vi "Poll Home Control.vi"(8 "error in (no error)":errorcluster, 11 "Cylinder.lvclass":refnum<class "Cylinder.lvclass">) -> ()   [LabVIEW 2015, in "cRIO-Carbondioxide.lvlib" / "CO2-Actor.lvlib" / "Cylinder.lvclass"]
uses:
  Cylinder.lvclass
  Cylinder.lvclass/Cylinder.ctl
  <vilib>/ActorFramework/Actor/Actor.lvclass/Actor.ctl
  <vilib>/ActorFramework/Message Enqueuer/Message Enqueuer.lvclass/Message Enqueuer.ctl
  Cylinder Messages/Run Msg/Run Msg.lvclass/Run Msg.ctl
  Cylinder Messages/Home Msg/Home Msg.lvclass/Home Msg.ctl
  <vilib>/ActorFramework/Actor/Read Self Enqueuer.vi
  <vilib>/ActorFramework/Message Enqueuer/Enqueue.vi
  <vilib>/ActorFramework/Message Enqueuer/Init from Existing Queue.vi
  <vilib>/ActorFramework/Message Priority Queue/Priority Enqueue.vi
  <vilib>/ActorFramework/Actor/Actor.lvclass
  <vilib>/ActorFramework/Message Enqueuer/Message Enqueuer.lvclass
  Interlocks/Interlock Chain/Interlock Chain.lvclass
  Cylinder Messages/Run Msg/Run Msg.lvclass
  Cylinder Messages/Home Msg/Home Msg.lvclass
  cRIO-CO2/cRIO-CO2.lvclass
  CO2 Actor/CO2 Actor.lvclass
panel:
  out "error out":errorcluster
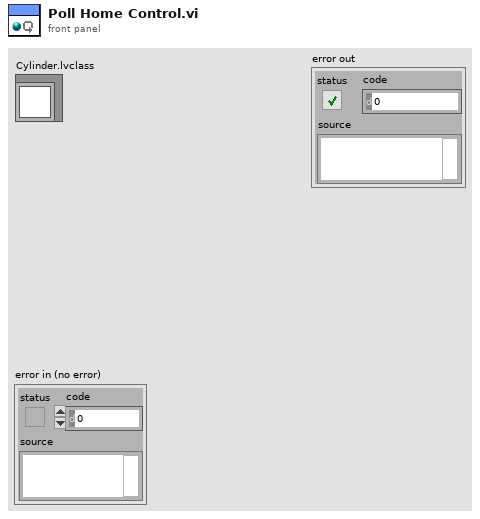
[diagram p1: front panel]
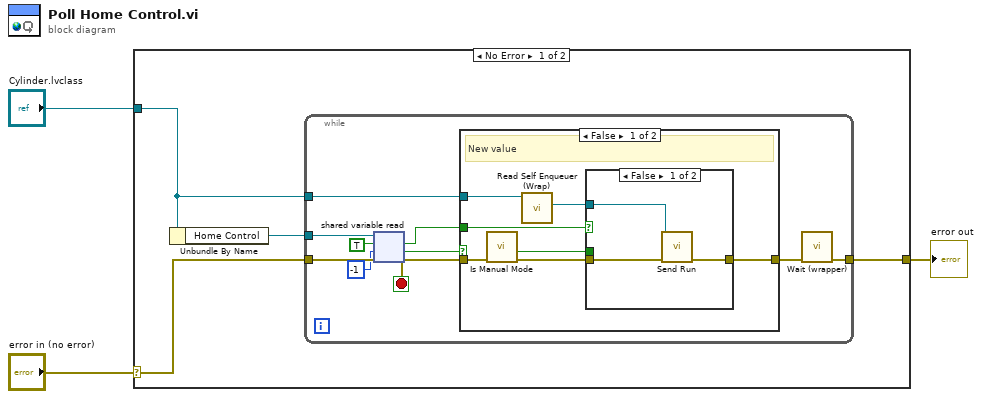
[diagram p0: block diagram]
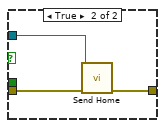
[diagram p2: hidden frame]
diagram:
  n1 = case shown="No Error" "error in (no error)" {
    selector: "error in (no error)" -> [w5 w32]
    tunnel: "Cylinder.lvclass" -> [w6 _]
    tunnel: [w4 w32] -> w1
    frame No Error {
      n2 = Unbundle By Name(w6) -> ("Home Control"=w7:refnum<k21>)
      n3 = while {
        tunnel: w7 -> [w17]
        tunnel: w5 -> [w16]
        tunnel: w6 -> [w10]
        tunnel: [w8] -> w4
        stop <- w11 stop-if-true
        n4 = shared-variable-read(w17, w16, TRUE, -1 ("timeout ms")) -> (w11:errorcluster, w9:bool, w12:bool)  [unwired: 2 out]
        n5 = case shown="False" w9 {
          tunnel: w12 -> [w21 _]
          tunnel: [w22 w31] -> w13
          tunnel: w11 -> [w24 w31]
          tunnel: w10 -> [w19 _]
          frame False {
            # "New value"
            n6 = call "Is Manual Mode.vi"("error in (no error)"=w24) -> ("error out"=w23:errorcluster, "Manual Mode?"=w20:bool)  [unwired: 9 in]
            n7 = call "Read Self Enqueuer (Wrap).vi"("CO2 Actor in"=w19) -> ("Actor Framework:Message Enqueuer"=w18:refnum<class "Message Enqueuer.lvclass">)  [unwired: 9 in, 1 out]
            n8 = case shown="False" w21 {
              tunnel: w23 -> [w27 w30]
              tunnel: [w26 w29] -> w22
              tunnel: w20 -> [_ _]
              tunnel: w18 -> [w25 w28]
              frame False {
                n9 = call "Send Run.vi"("error in (no error)"=w27, "Message Enqueuer"=w25) -> ("error out"=w26:errorcluster)  [unwired: 8 in, 1 out]
              }
              frame True {
                n10 = call "Send Home.vi"("error in (no error)"=w30, "Message Enqueuer"=w28) -> ("error out"=w29:errorcluster)  [unwired: 8 in, 1 out]
              }
            }
          }
          frame True {
            # "Timeout"
          }
        }
        n11 = call "Wait (wrapper).vi"("error in (no error)"=w13) -> ("error out"=w8:errorcluster)  [unwired: 10 in]
      }
    }
    frame Error {
    }
  }
  "error out" <- w1
